vi "Actor Core.vi"(8 "error in":errorcluster, 11 "Simulated Oscilloscope in":refnum<class "Simulated Oscilloscope.lvclass">) -> (0 "error out":errorcluster, 3 "Actor out":refnum<class "Actor.lvclass">)   [LabVIEW 2014, in "Simulated Oscilloscope.lvclass"]
doc: "(<B>Filename</B>: Actor Framework.lvlib:Actor.lvclass:Actor Core.vi)\n\nReceives messages to the actor, reacts to them, and initiates any error handling that may shut the actor down.\n\nDescendant classes may override this VI to append parallel tasks for the actor to complete while it handles messages. Overrides use the Call Parent Method node."
uses:
  Simulated Oscilloscope.lvclass
  <vilib>/ActorFramework/Actor/Actor.lvclass
  Params.ctl
  <vilib>/ActorFramework/Actor/Actor.lvclass/Actor.ctl
  <vilib>/ActorFramework/Message Enqueuer/Message Enqueuer.lvclass/Message Enqueuer.ctl
  Simulated Oscilloscope.lvclass/Simulated Oscilloscope.ctl
  Simulated Oscilloscope Messages/Write params Msg/Write params Msg.lvclass/Write params Msg.ctl
  Framework/Interfaces/Pipelined Actor/Pipelined Actor Messages/Do Main Action Msg/Do Main Action Msg.lvclass/Do Main Action Msg.ctl
  Framework/Model/Data/Data1D/Data1D.lvclass
  <vilib>/ActorFramework/Message Enqueuer/Init from Existing Queue.vi
  <vilib>/ActorFramework/Message Enqueuer/Enqueue.vi
  <vilib>/ActorFramework/Message Priority Queue/Priority Enqueue.vi
  <vilib>/ActorFramework/Message Enqueuer/Message Enqueuer.lvclass
  Simulated Oscilloscope Messages/Write params Msg/Write params Msg.lvclass
  Framework/Model/Data/AbstractData/AbstractData.lvclass
  Framework/Interfaces/Pipelined Actor/Pipelined Actor Messages/Do Main Action Msg/Do Main Action Msg.lvclass
  Framework/Hardware/ReadoutDevice/ReadoutDevice.lvclass
  Framework/Interfaces/Viewable Actor/Viewable Actor.lvclass
  Framework/Interfaces/Observable Actor/Observable Actor.lvclass
panel:
  out "isShow":bool=TRUE
  in  "Read":bool
  out "Stop":bool=TRUE
  in  "dt":dbl=0.1
  in  "Frequency":dbl=100.0
  in  "Noise Amplitude":dbl=2.0
  in  "Y Offset":dbl=2.0
  in  "X Offset":dbl=5.0
  in  "Ticks per frame":dbl=1000.0
  in  "Period":dbl=100.0
  in  "Amplitude":dbl=100.0
  out "Preview Graph":waveform(dbl)(graph)
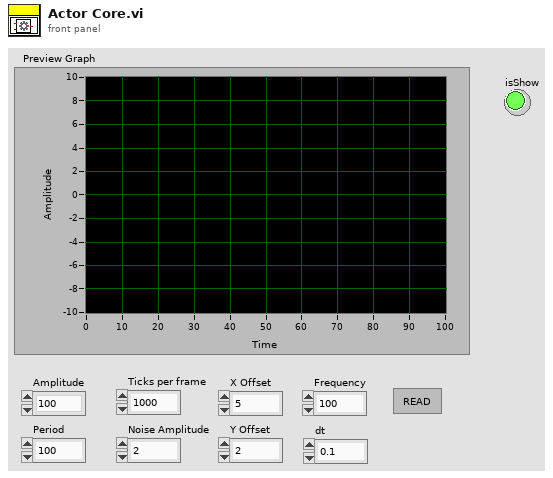
[diagram p1: front panel]
types:
  T1 = typedef "Simulated Oscilloscope.lvclass/Params.ctl" = cluster{"Amplitude":dbl, "Y Offset":dbl, "X Offset":dbl, "Period":dbl, "Ticks per frame":dbl, "Noise Amplitude":dbl, "dt":dbl}
  T2 = typedef "Observable Actor.lvlib/Observable Actor.lvclass/Observer.ctl" = refnum<queue>
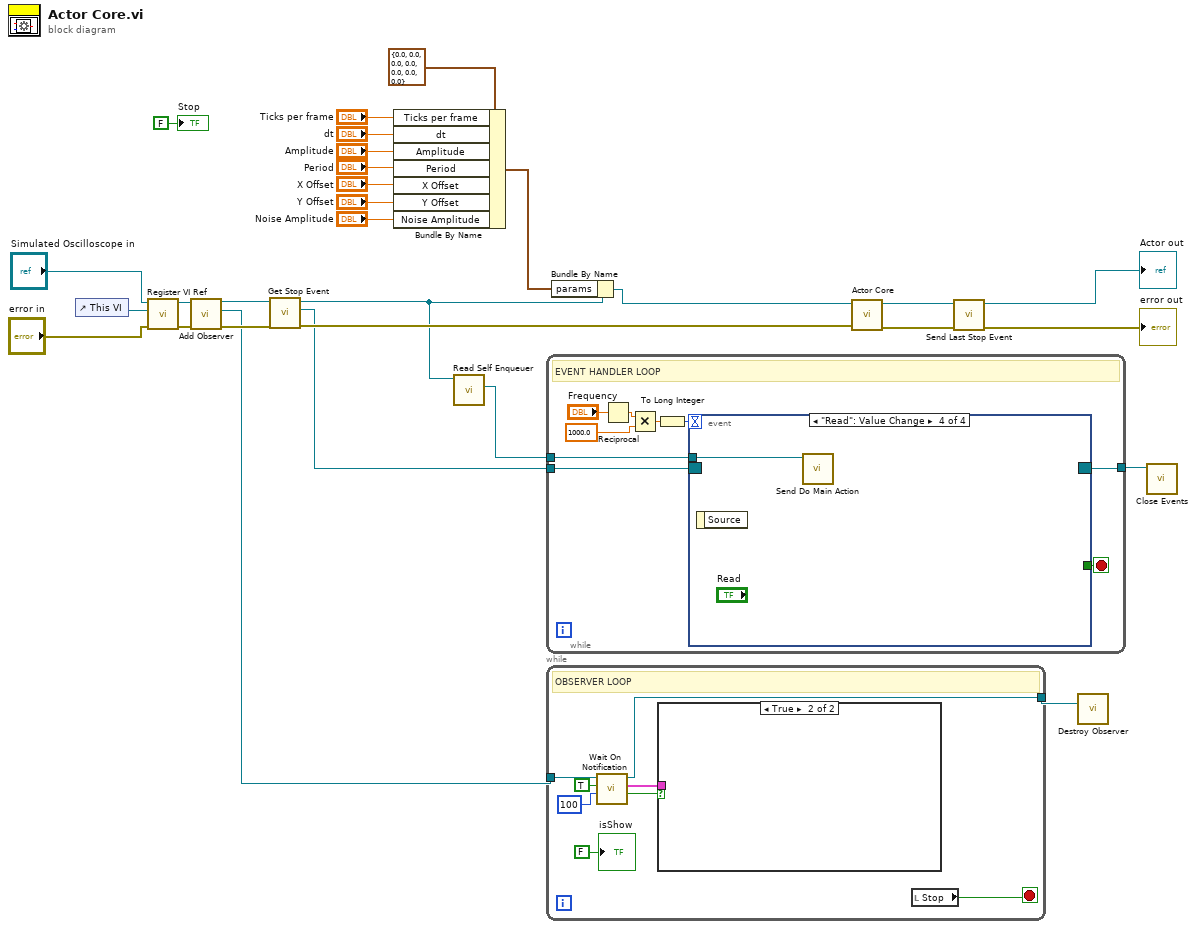
[diagram p0: block diagram]
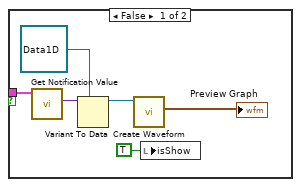
[diagram p2: hidden frame]
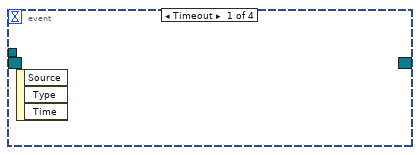
[diagram p3: hidden frame]
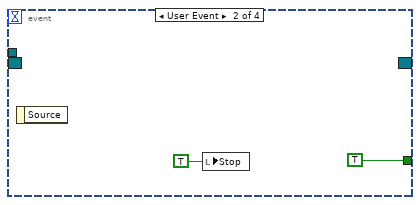
[diagram p4: hidden frame]
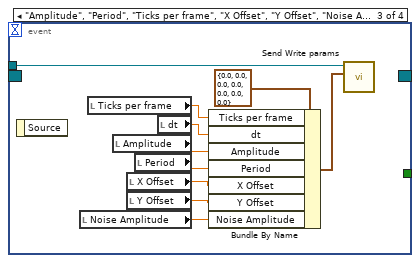
[diagram p5: hidden frame]
diagram:
  n1 = control-ref of="This VI"() -> (w26:refnum<vi>)
  n2 = call "Register VI Ref.vi"("error in (no error)"="error in", "VI ref"=w26, "Viewable Actor in"="Simulated Oscilloscope in") -> ("error out"=w22:errorcluster, "Viewable Actor out"=w23:refnum<class "Simulated Oscilloscope.lvclass">)  [unwired: 7 in]
  n3 = call-dynamic "Add Observer.vi"("error in (no error)"=w22, "Observable Actor in"=w23) -> ("error out"=w29:errorcluster, "new observer"=w21:T2, "Observable Actor out"=w20:refnum<class "Simulated Oscilloscope.lvclass">)  [unwired: 7 in]
  n4 = call-dynamic "Get Stop Event.vi"("error in (no error)"=w29, "Observable Actor in"=w20) -> ("error out"=w19:errorcluster, "Events"=w18:refnum<event-registration>, "Observable Actor out"=w2:refnum<class "Simulated Oscilloscope.lvclass">)  [unwired: 7 in]
  n5 = Bundle By Name(cluster=T1 {"Amplitude"=0.0, "Y Offset"=0.0, "X Offset"=0.0, "Period"=0.0, "Ticks per frame"=0.0, "Noise Amplitude"=0.0, "dt"=0.0} ("output"), "Ticks per frame"="Ticks per frame", "dt"="dt", "Amplitude"="Amplitude", "Period"="Period", "X Offset"="X Offset", "Y Offset"="Y Offset", "Noise Amplitude"="Noise Amplitude") -> (w3:T1)
  n6 = call <vilib>:"Read Self Enqueuer.vi"("Actor"=w2) -> ("Self Enqueuer"=w25:refnum<class "Message Enqueuer.lvclass">)  [unwired: 10 in]
  n7 = while {
    tunnel: w18 -> [w38]
    tunnel: w25 -> [w37]
    tunnel: [w36] -> w17
    stop <- w35 stop-if-true
    # "EVENT HANDLER LOOP"
    n8 = Reciprocal(x="Frequency") -> (1/x=w33:dbl)
    n9 = Multiply(x=w33, y=1000.0) -> (x*y=w31:dbl)
    n10 = To Long Integer(number=w31) -> (32bit integer=w30:i32)
    n11 = event shown="[3] \"Read\": Value Change" {
      selector: w38 -> [_ _ _ _]
      dyn-events: [_ _ _ _] -> w36
      timeout: w30 -> [_ _ _ _]
      tunnel: w37 -> [_ _ w50 w51]
      tunnel: [_ TRUE _ _] -> w35
      event Timeout {
        n12 = event-data() -> ()  [unwired: 1 in, 3 out]
      }
      event User Event {
        n13 = event-data() -> ()  [unwired: 1 in, 1 out]
        n14 = local write "Stop"(TRUE ("Stop")) -> ()
      }
      event "Amplitude", "Period", "Ticks per frame", "X Offset", "Y Offset", "Noise Amplitude", "Frequency", "dt": Value Change {
        n15 = event-data() -> ()  [unwired: 1 in, 1 out]
        n16 = local read "Noise Amplitude"() -> (w49:dbl)
        n17 = local read "Ticks per frame"() -> (w43:dbl)
        n18 = local read "Amplitude"() -> (w45:dbl)
        n19 = local read "X Offset"() -> (w47:dbl)
        n20 = local read "Y Offset"() -> (w48:dbl)
        n21 = local read "Period"() -> (w46:dbl)
        n22 = local read "dt"() -> (w44:dbl)
        n23 = Bundle By Name(cluster=T1 {"Amplitude"=0.0, "Y Offset"=0.0, "X Offset"=0.0, "Period"=0.0, "Ticks per frame"=0.0, "Noise Amplitude"=0.0, "dt"=0.0} ("output"), "Ticks per frame"=w43, "dt"=w44, "Amplitude"=w45, "Period"=w46, "X Offset"=w47, "Y Offset"=w48, "Noise Amplitude"=w49) -> (w41:T1)
        n24 = call "Send Write params.vi"("output"=w41, "Message Enqueuer"=w50) -> ()  [unwired: 8 in, 2 out]
      }
      event "Read": Value Change {
        n25 = event-data() -> ()  [unwired: 1 in, 1 out]
        n26 = call "Send Do Main Action.vi"("Message Enqueuer"=w51) -> ()  [unwired: 9 in, 2 out]
      }
    }
  }
  n27 = while {
    tunnel: w21 -> [w54]
    tunnel: [w53] -> w12
    stop <- w59 stop-if-true
    # "OBSERVER LOOP"
    n28 = call "Wait On Notification.vi"("timeout in ms (-1)"=100, "ignore previous (F)"=TRUE, "observer in"=w54) -> ("timed out?"=w55:bool, "notification"=w56:cluster{"value":variant, "name":string}, "observer out"=w53:T2)  [unwired: 5 in, 1 out]
    n29 = case shown="True" w55 {
      tunnel: w56 -> [w65 _]
      frame False {
        n30 = call "Get Notification Value.vi"("notification in"=w65) -> ("data"=w64:variant)  [unwired: 7 in, 1 out]
        n31 = Variant To Data(type=refnum<class "Data1D.lvclass"> refnum ("Data1D in"), Variant=w64) -> (data=w62:refnum<class "Data1D.lvclass">)  [unwired: 1 in, 1 out]
        n32 = call "Create Waveform.vi"("Data1D in"=w62) -> ("Waveform"=→"Preview Graph":waveform(dbl))  [unwired: 8 in, 2 out]
        n33 = local write "isShow"(TRUE ("isShow")) -> ()
      }
      frame True {
      }
    }
    n34 = local read "Stop"() -> (w59:bool)
    "isShow" <- FALSE ("Boolean")
  }
  n35 = Bundle By Name(cluster=w2, "params"=w3) -> (w1:refnum<class "Simulated Oscilloscope.lvclass">)
  n36 = call-parent "Actor Core.vi"("error in"=w19, "Actor in"=w1) -> ("error out"=w15:errorcluster, "Actor out"=w16:refnum<class "Actor.lvclass">)  [unwired: 8 in]
  n37 = call "Send Last Stop Event.vi"("error in (no error)"=w15, "Actor in"=w16) -> ("error out"=→"error out":errorcluster, "Actor  out"=→"Actor out":refnum<class "Actor.lvclass">)  [unwired: 8 in]
  n38 = call "Destroy Observer.vi"("observer in"=w12) -> ()  [unwired: 11 in]
  n39 = call "Close Events.vi"("events"=w17) -> ()  [unwired: 11 in]
  "Stop" <- FALSE ("Stop")
